vi "Write Init.vi"(8 "error in (no error)":errorcluster, 10 "Init":bool, 11 "Vapour Generator in":refnum<class "Vapour Generator.lvclass">) -> (0 "error out":errorcluster, 3 "Vapour Generator out":refnum<class "Vapour Generator.lvclass">)   [LabVIEW 2011, in "Vapour Generator.lvclass"]
uses:
  Vapour Generator.lvclass
  Vapour Generator.lvclass/Vapour Generator.ctl
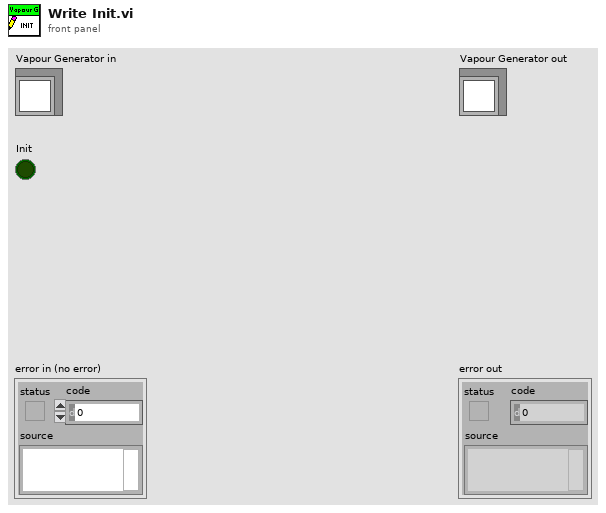
[diagram p1: front panel]
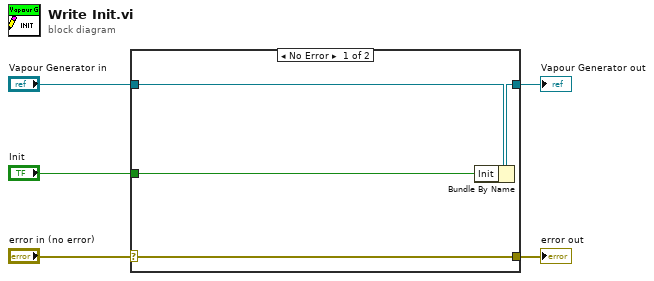
[diagram p0: block diagram]
diagram:
  n1 = case shown="No Error" "error in (no error)" {
    selector: "error in (no error)" -> [w9 w10]
    tunnel: [w9 w10] -> w4
    tunnel: [w7 w11] -> w2
    tunnel: "Vapour Generator in" -> [w8 w11]
    tunnel: "Init" -> [w6 _]
    frame No Error {
      n2 = Bundle By Name(cluster=w8, "Init"=w6) -> (w7:refnum<class "Vapour Generator.lvclass">)
    }
    frame Error {
    }
  }
  "error out" <- w4
  "Vapour Generator out" <- w2
